vi "Run Post-Section Hook.vi"(8 "Error In":errorcluster, 10 "Output In":string, 11 "Context In":refnum<class "Compiler.lvclass">) -> (0 "Error Out":errorcluster, 2 "Output Out":string, 3 "Context Out":refnum<class "Compiler.lvclass">)   [LabVIEW 2018, in "Toolkit.lvlib" / "Renderer.lvclass"]
uses:
  Renderer.lvclass
  Hooks/Render/Section/Section.lvclass
  Context/Compiler.lvclass
  Data/Datum/Datum.lvclass
  D:/Users/cfield/Code/Field R&D Services/Labstache/src/Toolkit/Hooks/Hook/Hook.lvclass
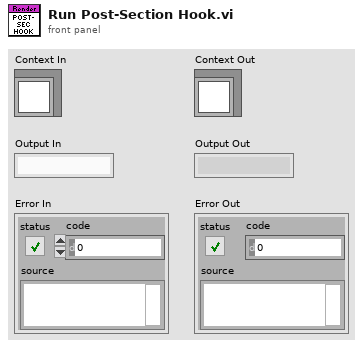
[diagram p1: front panel]
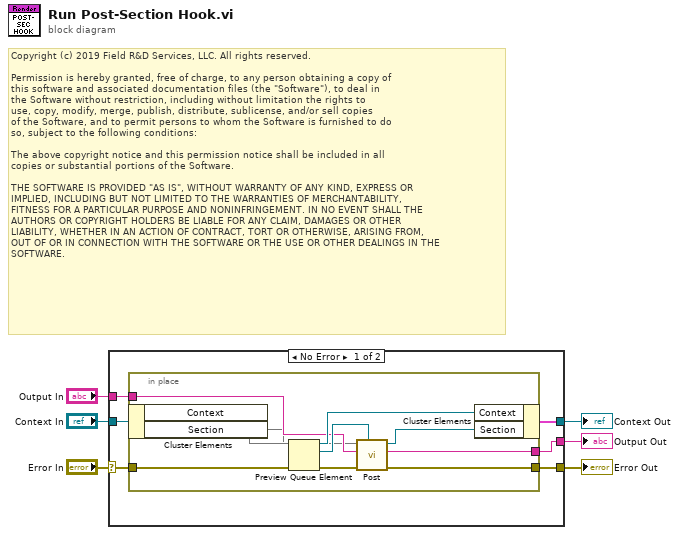
[diagram p0: block diagram]
diagram:
  # "Copyright (c) 2019 Field R&D Services, LLC. All rights reserved.\n\nPermission is hereby granted, free of charge, to any person obtaining a copy of\nthis software and associated documentation files (the \"Software\"), to deal in\nthe Software without restriction, including without limitation the rights to\nuse, copy, modify, merge, publish, distribute, sublicense, and/or sell copies\nof the Software, and to permit persons to whom the Software is furnished to do\nso, subject to the following conditions:\n\nThe above copyright notice and this permission notice shall be included in all\ncopies or substantial portions of the Software.\n\nTHE SOFTWARE IS PROVIDED \"AS IS\", WITHOUT WARRANTY OF ANY KIND, EXPRESS OR\nIMPLIED, INCLUDING BUT NOT LIMITED TO THE WARRANTIES OF MERCHANTABILITY,\nFITNESS FOR A PARTICULAR PURPOSE AND NONINFRINGEMENT. IN NO EVENT SHALL THE\nAUTHORS OR COPYRIGHT HOLDERS BE LIABLE FOR ANY CLAIM, DAMAGES OR OTHER\nLIABILITY, WHETHER IN AN ACTION OF CONTRACT, TORT OR OTHERWISE, ARISING FROM,\nOUT OF OR IN CONNECTION WITH THE SOFTWARE OR THE USE OR OTHER DEALINGS IN THE\nSOFTWARE."
  n1 = case shown="No Error" "Error In" {
    selector: "Error In" -> [w12 w24]
    tunnel: "Context In" -> [w9 w25]
    tunnel: [w11 w25] -> w4
    tunnel: [w10 w24] -> w3
    tunnel: "Output In" -> [w8 w23]
    tunnel: [w7 w23] -> w1
    frame No Error {
      n2 = in-place {
        in-place-border: w12 -> [w18]
        in-place-border: [w22] -> w10
        in-place-border: [w21] -> w7
        in-place-border: w8 -> [w15]
        n3 = in-place-cluster #1(w9) -> ("Context"=w20, "Section"=w14)
        n4 = Preview Queue Element(queue=w20, error in (no error)=w18) -> (queue out=w19:refnum<queue>, element=w16:refnum<class "Datum.lvclass">, error out=w17:errorcluster)  [unwired: 1 in, 1 out]
        n5 = call-dynamic "Post.vi"("Datum"=w16, "Error In"=w17, "Output In"=w15, "Render Section In"=w14) -> ("Error Out"=w22:errorcluster, "Output Out"=w21:string, "Render Section Out"=w13:refnum<class "Section.lvclass">)  [unwired: 5 in]
        n6 = in-place-cluster #1("Context"=w19, "Section"=w13) -> (w11:cluster{})
      }
    }
    frame Error {
    }
  }
  "Context Out" <- w4
  "Error Out" <- w3
  "Output Out" <- w1
